vi "Add Through Points 2.vi"(4 "Side":T1=enum."right", 8 "Use":bool=TRUE, 11 "Goal":cluster{"Label":string, "Goal":dbl[]}) -> (3 "Goal":cluster{"Label":string, "Goal":dbl[]})   [LabVIEW 2013]
uses:
  ROS/Code/SubVIs/BaxterSide.ctl
  Arm Globals.vi
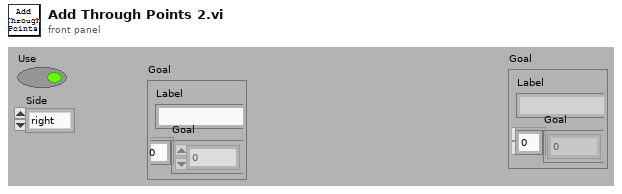
[diagram p1: front panel]
types:
  T1 = typedef "BaxterSide.ctl" = enum16{"left", "right"}
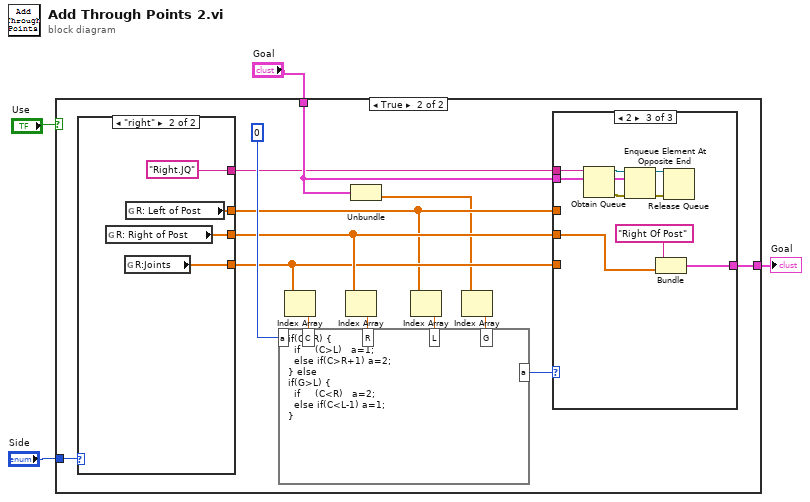
[diagram p0: block diagram]
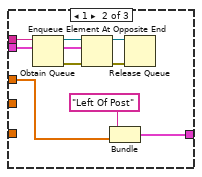
[diagram p4: hidden frame]
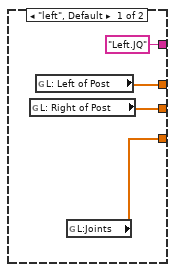
[diagram p5: hidden frame]
diagram:
  n1 = case shown="True" "Use" {
    tunnel: "Side" -> [_ w19]
    tunnel: [w5 w7] -> w1
    tunnel: "Goal" -> [w5 w8]
    frame False {
    }
    frame True {
      n2 = case shown="\"right\"" w19 {
        tunnel: [w39 w43] -> w11
        tunnel: [w42 w46] -> w10
        tunnel: [w41 w45] -> w12
        tunnel: ["Left.JQ" "Right.JQ"] -> w6
        frame "left", Default {
          n3 = global read "Arm Globals.vi" "L: Right of Post"() -> (w41:dbl[])
          n4 = global read "Arm Globals.vi" "L: Left of Post"() -> (w42:dbl[])
          n5 = global read "Arm Globals.vi" "L:Joints"() -> (w39:dbl[])
        }
        frame "right" {
          n6 = global read "Arm Globals.vi" "R: Right of Post"() -> (w45:dbl[])
          n7 = global read "Arm Globals.vi" "R:Joints"() -> (w43:dbl[])
          n8 = global read "Arm Globals.vi" "R: Left of Post"() -> (w46:dbl[])
        }
      }
      n9 = Index Array(array=w11) -> (element=w16:dbl)  [unwired: 1 in]
      n10 = Index Array(array=w12) -> (element=w15:dbl)  [unwired: 1 in]
      n11 = Unbundle(w8) -> ("Goal"=w9:dbl[])  [unwired: 1 out]
      n12 = Index Array(array=w10) -> (element=w17:dbl)  [unwired: 1 in]
      n13 = Index Array(array=w9) -> (element=w18:dbl)  [unwired: 1 in]
      n14 = formula code="if(G<R) {\n  if     (C>L)   a=1;\n  else if(C>R+1) a=2;\n} else \nif(G>L) {\n  if     (C<R)   a=2;\n  else if(C<L-1) a=1;\n}"("G"=w18, "L"=w17, "C"=w16, "R"=w15, "a"=0) -> ("a"=w13:i32)
      n15 = case shown="2" w13 {
        tunnel: w12 -> [_ _ w30]
        tunnel: w11 -> [_ _ _]
        tunnel: w10 -> [_ w28 _]
        tunnel: w8 -> [w20 w22 w32]
        tunnel: [w20 w27 w37] -> w7
        tunnel: w6 -> [_ w21 w31]
        frame 0, Default {
        }
        frame 1 {
          n16 = Obtain Queue(name (unnamed)=w21, element data type=w22) -> (queue out=w23:refnum<queue>, error out=w24:errorcluster)  [unwired: 3 in, 1 out]
          n17 = Enqueue Element At Opposite End(queue=w23, element=w22, error in (no error)=w24) -> (queue out=w25:refnum<queue>, error out=w26:errorcluster)  [unwired: 1 in, 1 out]
          n18 = Bundle("Left Of Post", "R: Left of Post"=w28) -> (w27:cluster{string, "R: Left of Post":dbl[]})  [unwired: 1 in]
          n19 = Release Queue(queue=w25, error in (no error)=w26) -> ()  [unwired: 1 in, 3 out]
        }
        frame 2 {
          n20 = Obtain Queue(name (unnamed)=w31, element data type=w32) -> (queue out=w33:refnum<queue>, error out=w34:errorcluster)  [unwired: 3 in, 1 out]
          n21 = Enqueue Element At Opposite End(queue=w33, element=w32, error in (no error)=w34) -> (queue out=w35:refnum<queue>, error out=w36:errorcluster)  [unwired: 1 in, 1 out]
          n22 = Bundle("Right Of Post", "R: Right of Post"=w30) -> (w37:cluster{string, "R: Right of Post":dbl[]})  [unwired: 1 in]
          n23 = Release Queue(queue=w35, error in (no error)=w36) -> ()  [unwired: 1 in, 3 out]
        }
      }
    }
  }
  "Goal" <- w1
